vi "QuickDrop Parse Plugin Variant.vi"(0 "QDKS Variant in":variant) -> (4 "QD Launch VI Panel?":bool, 6 "Project VI Path":path, 8 "Palette Object Name":string)   [LabVIEW 2017]
uses:
  <vilib>/Utility/QuickDropSupport/QuickDrop Plugin Data ver1.ctl
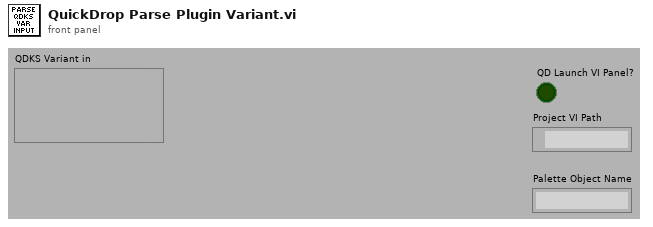
[diagram p1: front panel]
types:
  T1 = typedef "QuickDrop Plugin Data ver1.ctl" = cluster{"FP.IsFrontMost?":bool, "Project VI Path":path, "Palette Object Name":string}
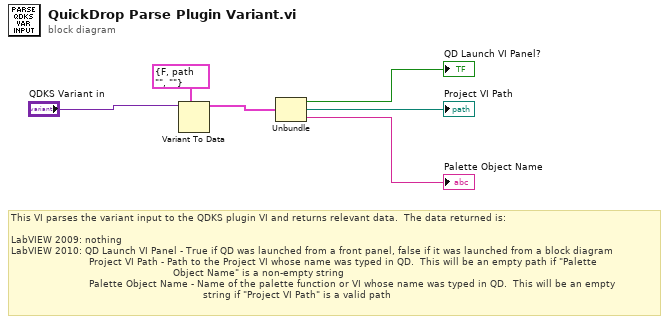
[diagram p0: block diagram]
diagram:
  # "This VI parses the variant input to the QDKS plugin VI and returns relevant data.  The data returned is:\n\nLabVIEW 2009: nothing\nLabVIEW 2010: QD Launch VI Panel - True if QD was launched from a front panel, false if it was launched from a block diagram\n                          Project VI Path - Path to the Project VI whose name was typed in QD.  This will be an empty path if \"Palette\n                                                      Object Name\" is a non-empty string\n                          Palette Object Name - Name of the palette function or VI whose name was typed in QD.  This will be an empty\n                                                                string if \"Project VI Path\" is a valid path"
  n1 = Variant To Data(type=T1 {"FP.IsFrontMost?"=FALSE, "Project VI Path"=path "", "Palette Object Name"=""} ("Quick Drop Plugin Data"), Variant="QDKS Variant in") -> (data=w4:T1)  [unwired: 1 in, 1 out]
  n2 = Unbundle(w4) -> ("FP.IsFrontMost?"=→"QD Launch VI Panel?":bool, "Project VI Path"=→"Project VI Path":path, "Palette Object Name"=→"Palette Object Name":string)
